vi "Get Parameter Value.vi"(6 "Clear Null":bool=TRUE, 10 "Parameter Name":string, 11 "JSON":string) -> (1 "Found":bool, 2 "Parameter Value":string, 3 "Remaining JSON":string, 4 "Null":bool)   [LabVIEW 2015, in "NI_JSON Parsing.lvlib"]
uses:
  NI_JSON Parsing.lvlib
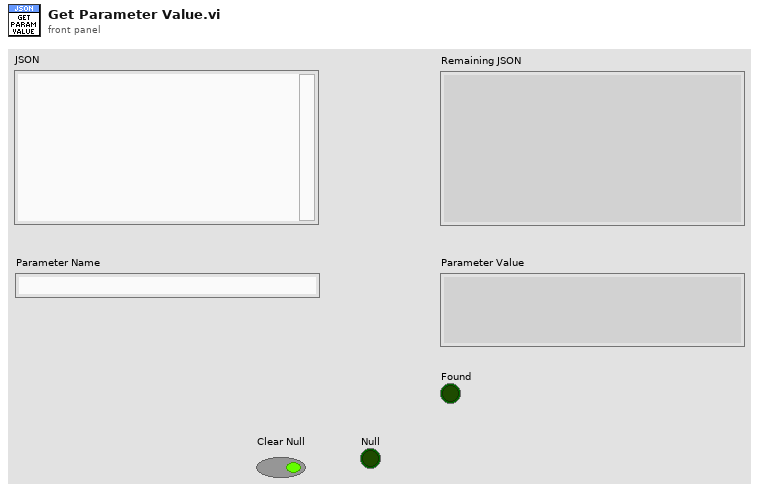
[diagram p1: front panel]
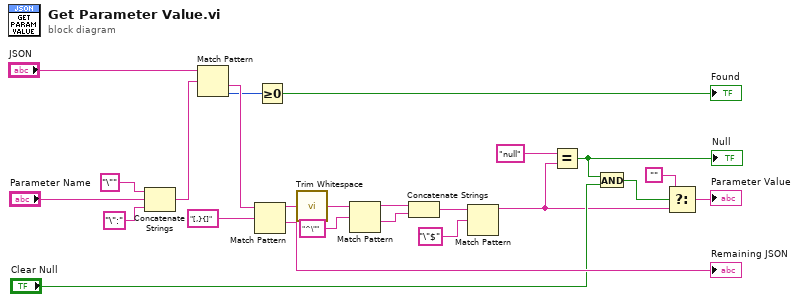
[diagram p0: block diagram]
diagram:
  n1 = Concatenate Strings("\"" ("string"), "Parameter Name", "\":" ("string")) -> (w18:string)
  n2 = Match Pattern(string="JSON", regular expression=w18) -> (after substring=w22:string, offset past match=w9:i32)  [unwired: 1 in, 2 out]
  n3 = Match Pattern(string=w22, regular expression="[,}{]") -> (before substring=w20:string, after substring=→"Remaining JSON":string)  [unwired: 1 in, 2 out]
  n4 = Greater Or Equal To 0?(x=w9) -> (x >= 0?=→"Found":bool)
  n5 = call <vilib>:"Trim Whitespace.vi"("string"=w20) -> ("trimmed string"=w15:string)  [unwired: 1 in]
  n6 = Match Pattern(string=w15, regular expression="^\"") -> (before substring=w13:string, after substring=w12:string)  [unwired: 1 in, 2 out]
  n7 = Concatenate Strings(w13, w12) -> (w11:string)
  n8 = Match Pattern(string=w11, regular expression="\"$") -> (before substring=w4:string)  [unwired: 1 in, 3 out]
  n9 = Equal?(x="null", y=w4) -> (x = y?=w5:bool)
  "Null" <- w5
  n10 = And(x=w5, y="Clear Null") -> (x .and. y?=w2:bool)
  n11 = Select(t="", s=w2, f=w4) -> (s? t:f=→"Parameter Value":string)
